vi "6509 Control Outputs.vi"(1 "error in (no error)":errorcluster, 2 "Enable Output":bool, 3 "Enum":T1(ring)) -> (0 "error out":errorcluster)   [LabVIEW 2014]
panel:
  in  "data":bool[](array[boolean])
  # "Pos 4"
  # "pos 5"
  # "Pos 10"
  # "Pos 11"
  # "Pos 12"
  # "Pos 13"
  # "Pos 14"
  # "Pos 15"
  # "Pos 7"
  # "Pos 0"
  # "Pos 1"
  # "Pos 2"
  # "Pos 3"
  # "Pos 6"
  # "Pos 8"
  # "Pos 9"
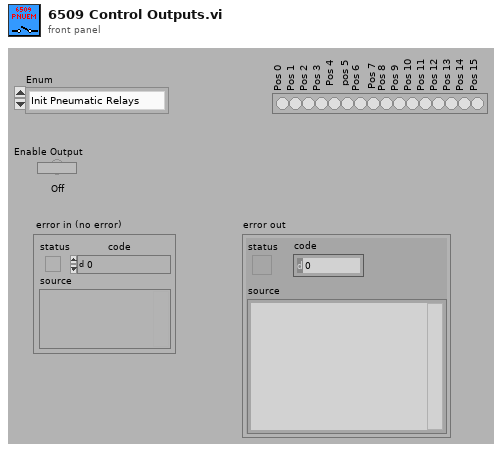
[diagram p1: front panel]
types:
  T1 = enum16{"Init Pneumatic Relays", "P5.0", "P5.1", "P5.2", "P5.3", "P5.4", "P5.5", "P5.6", "P5.7", "P2.6", "P2.7"}
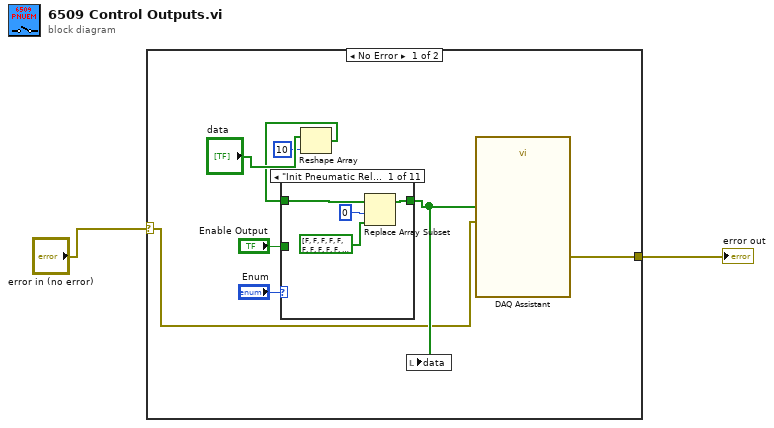
[diagram p0: block diagram]
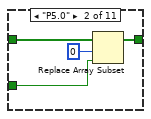
[diagram p2: hidden frame]
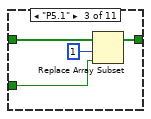
[diagram p3: hidden frame]
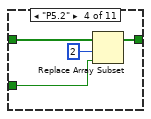
[diagram p4: hidden frame]
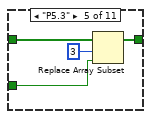
[diagram p5: hidden frame]
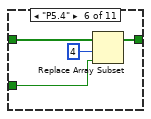
[diagram p6: hidden frame]
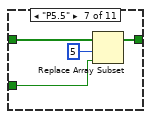
[diagram p7: hidden frame]
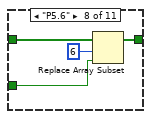
[diagram p8: hidden frame]
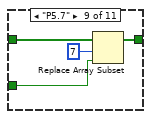
[diagram p9: hidden frame]
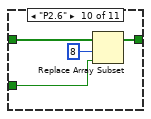
[diagram p10: hidden frame]
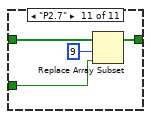
[diagram p11: hidden frame]
diagram:
  n1 = case shown="No Error" "error in (no error)" {
    selector: "error in (no error)" -> [w3 w55]
    tunnel: [w9 w55] -> w2
    frame No Error {
      n2 = Reshape Array("data", 10 ("dimension size")) -> (w5:bool[])
      n3 = case shown="\"Init Pneumatic Relays\", Default" "Enum" {
        tunnel: "Enable Output" -> [_ w18 w20 w24 w28 w32 w36 w40 w44 w48 w52]
        tunnel: w5 -> [w14 w17 w21 w25 w29 w33 w37 w41 w45 w49 w53]
        tunnel: [w12 w15 w19 w23 w27 w31 w35 w39 w43 w47 w51] -> w4
        frame "Init Pneumatic Relays", Default {
          n4 = Replace Array Subset(array=w14, new element=bool[] [FALSE, FALSE, FALSE, FALSE, FALSE, FALSE, FALSE, FALSE, FALSE, FALSE, FALSE, FALSE, FALSE, FALSE, FALSE, FALSE, FALSE, FALSE, FALSE, FALSE, FALSE, FALSE, FALSE, FALSE] ("data 2"), index=0) -> (w12:bool[])
        }
        frame "P5.0" {
          n5 = Replace Array Subset(array=w17, new element=w18, index=0) -> (w15:bool[])
        }
        frame "P5.1" {
          n6 = Replace Array Subset(array=w21, new element=w20, index=1) -> (w19:bool[])
        }
        frame "P5.2" {
          n7 = Replace Array Subset(array=w25, new element=w24, index=2) -> (w23:bool[])
        }
        frame "P5.3" {
          n8 = Replace Array Subset(array=w29, new element=w28, index=3) -> (w27:bool[])
        }
        frame "P5.4" {
          n9 = Replace Array Subset(array=w33, new element=w32, index=4) -> (w31:bool[])
        }
        frame "P5.5" {
          n10 = Replace Array Subset(array=w37, new element=w36, index=5) -> (w35:bool[])
        }
        frame "P5.6" {
          n11 = Replace Array Subset(array=w41, new element=w40, index=6) -> (w39:bool[])
        }
        frame "P5.7" {
          n12 = Replace Array Subset(array=w45, new element=w44, index=7) -> (w43:bool[])
        }
        frame "P2.6" {
          n13 = Replace Array Subset(array=w49, new element=w48, index=8) -> (w47:bool[])
        }
        frame "P2.7" {
          n14 = Replace Array Subset(array=w53, new element=w52, index=9) -> (w51:bool[])
        }
      }
      n15 = local write "data"(w4) -> ()
      n16 = call "DAQ Assistant"("data"=w4, "error in"=w3) -> ("error out"=w9:errorcluster)  [unwired: 16 in, 1 out]
    }
    frame Error {
    }
  }
  "error out" <- w2
